vi "3D Robot Frame.vi"(2 "name":string) -> (0 "robot frame":refnum<vi>)   [LabVIEW 2011]
uses:
  Robot Parameters/Robot Parameters.vi
  <vilib>/picture/3D Picture Control/NI_3D Picture Control.lvlib
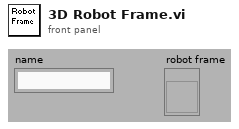
[diagram p1: front panel]
types:
  T1 = cluster{"Red":sgl, "Green":sgl, "Blue":sgl, "Alpha":sgl}
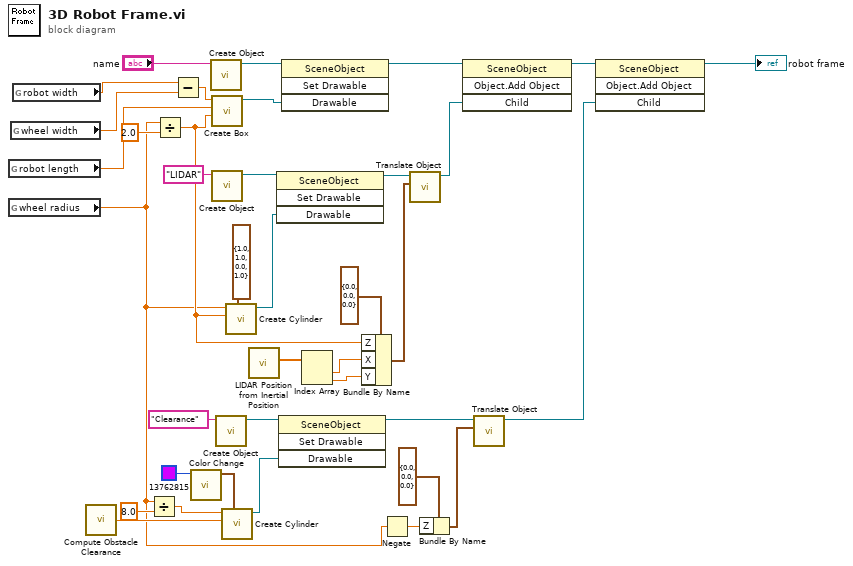
[diagram p0: block diagram]
diagram:
  n1 = global read "Robot Parameters.vi" "robot length"() -> (w2:dbl)
  n2 = global read "Robot Parameters.vi" "wheel radius"() -> (w1:dbl)
  n3 = global read "Robot Parameters.vi" "wheel width"() -> (w3:dbl)
  n4 = global read "Robot Parameters.vi" "robot width"() -> (w4:dbl)
  n5 = call "Compute Obstacle Clearance.vi"() -> ("obstacle clearance (m)"=w18:dbl)  [unwired: 1 in]
  n6 = Divide(x=w1, y=8.0) -> (x/y=w16:dbl)
  n7 = Divide(x=w1, y=2.0) -> (x/y=w27:dbl)
  n8 = Subtract(x=w4, y=w3) -> (x-y=w33:dbl)
  n9 = call <vilib>:"Color Change.vi"("Color"=u32 13762815) -> ("RGBA"=w5:cluster{"R":sgl, "G":sgl, "B":sgl, "A":sgl})  [unwired: 10 in]
  n10 = call <vilib>:"Create Object.vi"("Name"="name") -> ("Scene:New Object"=w34:refnum<vi>)  [unwired: 1 in, 9 out]
  n11 = call <vilib>:"Create Box.vi"("Length Z"=w27, "Length Y"=w2, "Length X"=w33) -> ("New Box Refnum"=w35:refnum<vi>)  [unwired: 1 in, 7 out]
  n12 = call <vilib>:"Create Object.vi"("Name"="LIDAR") -> ("Scene:New Object"=w32:refnum<vi>)  [unwired: 1 in, 9 out]
  n13 = call <vilib>:"Create Object.vi"("Name"="Clearance") -> ("Scene:New Object"=w19:refnum<vi>)  [unwired: 1 in, 9 out]
  n14 = call <vilib>:"Create Cylinder.vi"("Color"=w5, "Radius"=w18, "Height"=w16) -> ("New Cylinder Refnum"=w15:refnum<vi>)  [unwired: 1 in, 7 out]
  n15 = call <vilib>:"Create Cylinder.vi"("Color"=T1 {"Red"=1.0, "Green"=1.0, "Blue"=0.0, "Alpha"=1.0}, "Radius"=w27, "Height"=w1) -> ("New Cylinder Refnum"=w30:refnum<vi>)  [unwired: 1 in, 7 out]
  n16 = call "LIDAR Position from Inertial Position.vi"() -> ("LIDAR X, Y, Theta"=w9:dbl[])  [unwired: 11 in]
  n17 = invoke class="SceneObject" method="Set Drawable"(reference=w32, "Drawable"=w30) -> (reference out=w29:refnum<vi>)  [unwired: 2 in, 3 out]
  n18 = invoke class="SceneObject" method="Set Drawable"(reference=w19, "Drawable"=w15) -> (reference out=w14:refnum<vi>)  [unwired: 2 in, 3 out]
  n19 = invoke class="SceneObject" method="Set Drawable"(reference=w34, "Drawable"=w35) -> (reference out=w25:refnum<vi>)  [unwired: 2 in, 3 out]
  n20 = Index Array(array=w9) -> (element #1=w8:dbl, element #2=w7:dbl)  [unwired: 2 in]
  n21 = Bundle By Name(cluster=cluster{"X":sgl, "Y":sgl, "Z":sgl} {"X"=0.0, "Y"=0.0, "Z"=0.0} ("Translation"), "Z"=w27, "X"=w8, "Y"=w7) -> (w26:cluster{"X":sgl, "Y":sgl, "Z":sgl})
  n22 = Negate(x=w1) -> (-x=w12:dbl)
  n23 = call <vilib>:"Translate Object.vi"("Translation"=w26, "Scene.Object In"=w29) -> ("Scene.Object Out"=w24:refnum<vi>)  [unwired: 1 in, 8 out]
  n24 = Bundle By Name(cluster=cluster{"X":sgl, "Y":sgl, "Z":sgl} {"X"=0.0, "Y"=0.0, "Z"=0.0} ("Translation"), "Z"=w12) -> (w11:cluster{"X":sgl, "Y":sgl, "Z":sgl})
  n25 = invoke class="SceneObject" method="Object.Add Object"(reference=w25, "Child"=w24) -> (reference out=w22:refnum<vi>)  [unwired: 2 in, 3 out]
  n26 = call <vilib>:"Translate Object.vi"("Translation"=w11, "Scene.Object In"=w14) -> ("Scene.Object Out"=w10:refnum<vi>)  [unwired: 1 in, 8 out]
  n27 = invoke class="SceneObject" method="Object.Add Object"(reference=w22, "Child"=w10) -> (reference out=→"robot frame":refnum<vi>)  [unwired: 2 in, 3 out]
